vi "To ASCII Code.vi"   [LabVIEW 2016]
doc: "Takes in a String or a Float and convert it to an array ASCII code"
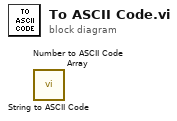
[diagram p0: block diagram]
diagram:
  n1 = call "String to ASCII Code.vi"() -> ()  [unwired: 10 in, 2 out]
  n2 = call "Number to ASCII Code Array.vi"() -> ()  [unwired: 10 in, 2 out]
